vi "Parte2_Medicion remota.vi"() -> ()   [LabVIEW 2020]
uses:
  <vilib>/httpClient/PUTBuffer.vi
  <vilib>/httpClient/LabVIEWHTTPClient.lvlib
panel:
  out "body":string
  out "headers":string
  out "error out":errorcluster
  in  "Rele":bool
  in  "Accionamiento":dbl(knob) scale=0.0..10.0
  in  "stop":bool
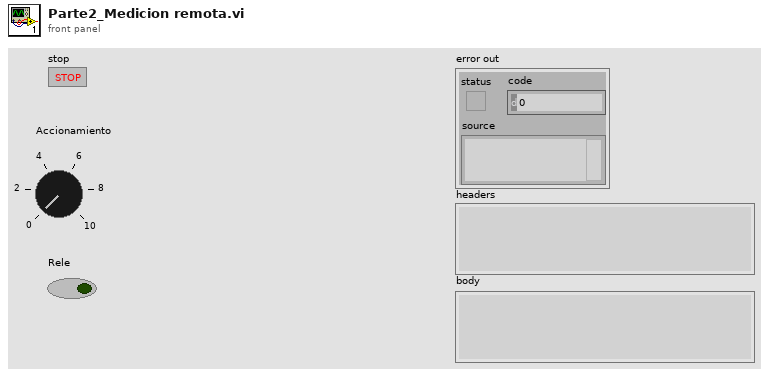
[diagram p1: front panel]
types:
  T1 = cluster{"Accionamineto ":dbl, "Data":string, "Hora":string, "Rele":bool}
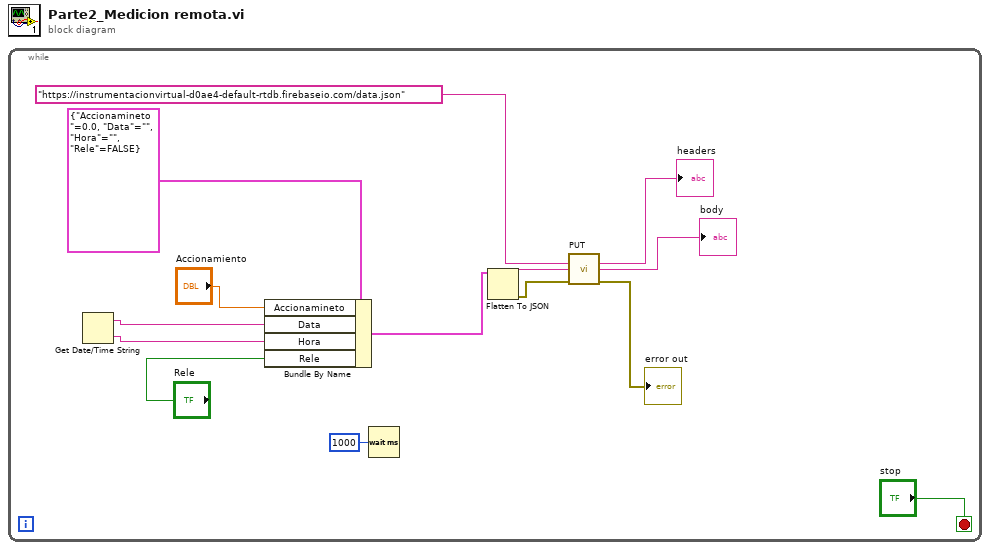
[diagram p0: block diagram]
diagram:
  n1 = while {
    stop <- "stop" stop-if-true
    n2 = Get Date/Time String() -> (date string=w10:string, time string=w9:string)  [unwired: 3 in]
    n3 = Bundle By Name(cluster=T1 {"Accionamineto "=0.0, "Data"="", "Hora"="", "Rele"=FALSE}, "Accionamineto"="Accionamiento", "Data"=w10, "Hora"=w9, "Rele"="Rele") -> (w8:T1)
    n4 = Wait (ms)(milliseconds to wait=u32 1000) -> ()  [unwired: 1 out]
    n5 = Flatten To JSON(anything=w8) -> (JSON string=w7:string, 11:w5:errorcluster)  [unwired: 2 in]
    n6 = call-poly <vilib>:"PUT.vi"("url"="https://instrumentacionvirtual-d0ae4-default-rtdb.firebaseio.com/data.json", "buffer"=w7, "error in (no error)"=w5) -> ("headers"=→"headers":string, "body"=→"body":string, "error out"=→"error out":errorcluster)  [unwired: 9 in, 1 out]
  }
